vi "Initialize.vi"(8 "error in (no error)":errorcluster, 11 "MeasurementServiceV2 in":refnum<class "MeasurementServiceV2.lvclass">) -> (0 "error out":errorcluster, 3 "MeasurementServiceV2 out":refnum<class "MeasurementServiceV2.lvclass">)   [LabVIEW 2020, in "MeasurementLink Measurement Server.lvlib" / "MeasurementServiceV2.lvclass"]
uses:
  MeasurementServiceV2.lvclass
  MeasurementLink Measurement Service V2_server/RPC Service/MeasurementService/MeasurementService.lvclass
  MeasurementServiceV2.lvclass/MeasurementServiceV2.ctl
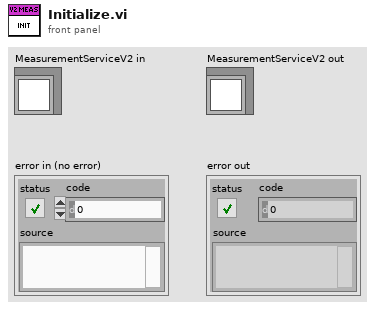
[diagram p1: front panel]
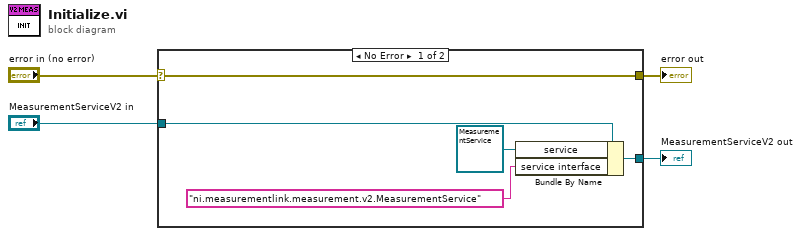
[diagram p0: block diagram]
diagram:
  n1 = case shown="No Error" "error in (no error)" {
    selector: "error in (no error)" -> [w9 w10]
    tunnel: [w9 w10] -> w3
    tunnel: "MeasurementServiceV2 in" -> [w8 w11]
    tunnel: [w6 w11] -> w1
    frame No Error {
      n2 = Bundle By Name(cluster=w8, "service"=refnum<class "MeasurementService.lvclass"> refnum, "service interface"="ni.measurementlink.measurement.v2.MeasurementService") -> (w6:refnum<class "MeasurementServiceV2.lvclass">)
    }
    frame Error {
    }
  }
  "MeasurementServiceV2 out" <- w1
  "error out" <- w3
